vi "DFD Filter Array.vi"(7 "init (F)":bool, 8 "error in (no error)":errorcluster, 10 "filters":T1[](array[typedef]) {"mSRate_QSettings"."source" items=["Coef a/k"=0, "Coef b/v"=7, "Input"=1, "Output"=2, "Multiplicand"=3, "Product"=4, "Sum"=5, "Delay"=6, "Gain"=8]}, 11 "signal in":waveform(dbl)[](array[waveform])) -> (0 "error out":errorcluster, 3 "signal out":waveform(dbl)[](array[waveform]))   [LabVIEW 2019, in "Instrument.Lockin.lvlib" / "Instrument.DAQ.lvclass"]
uses:
  Instrument.DAQ.lvclass
  <vilib>/addons/Digital Filter Design/NI_DigFilterLicensed.lvlib
  <vilib>/addons/Digital Filter Design/NI_DigFilter_Process.lvlib
  <vilib>/addons/Digital Filter Design/Process.llb/DFD Filtering with State (Wfm).vi
  <vilib>/addons/Digital Filter Design/_Objects.llb/DFD Filter Structure Type Selector.ctl
  <vilib>/addons/Digital Filter Design/_Objects.llb/DFD Filter Coef.ctl
  <vilib>/addons/Digital Filter Design/_Objects.llb/dfd_Internal Quantization Srcs.ctl
  <vilib>/addons/Digital Filter Design/_Objects.llb/dfd_Internal Quantization Settings.ctl
  <vilib>/addons/Digital Filter Design/_Objects.llb/DFD Coef Norm Type.ctl
  <vilib>/addons/Digital Filter Design/_Objects.llb/DFD Filter Obj.ctl
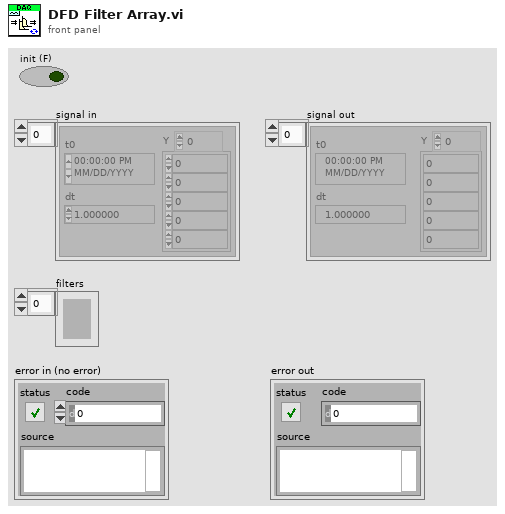
[diagram p1: front panel]
types:
  T1 = typedef "NI_DigFilterLicensed.lvlib/DFD Filter Obj.ctl" = cluster{"mSRate_Fs":dbl, "mSRate_Version":string, "mSRate_Comments":string, "mSRate_OrgCoef":T2, "mSRate_CurCoef":T2, "mSRate_Quantized?":bool, "mSRate_QCoef":T2, "mSRate_QSettings":T4[], "mSRate_Order":i32, "mSRate_Scaling":cluster{"mSRate_ScaleByPowerOf2?":bool, "mSRate_ScaleType":T6}}
  T2 = typedef "NI_DigFilterLicensed.lvlib/DFD Filter Coef.ctl" = cluster{"type":T3, "gain":dbl, "coef a (k)":dbl[], "coef b (v)":dbl[]}
  T3 = typedef "NI_DigFilterLicensed.lvlib/DFD Filter Structure Type Selector.ctl" = enum16{"Undefined", "FIR Direct Form", "FIR Direct Form Transposed", "FIR Symmetric", "FIR Antisymmetric", "IIR Direct Form I", "IIR Direct Form I Transposed", "IIR Direct Form II", "IIR Direct Form II Transposed", "IIR Cascaded Second Order Sections Form I", "IIR Cascaded Second Order Sections Form I Transposed", "IIR Cascaded Second Order Sections Form II", "IIR Cascaded Second Order Sections Form II Transposed", "Lattice Allpass (basic sections)", "Lattice Allpass (one multiplier sections)", "Lattice Allpass (normalized sections)", "Lattice AR (basic sections)", "Lattice AR (one multiplier sections)", "Lattice AR (normalized sections)", "Lattice MA (minimum phase)", "Lattice MA (maximum phase)", "Lattice ARMA (basic sections)", "Lattice ARMA (one multiplier sections)", "Lattice ARMA (normalized sections)"}
  T4 = typedef "NI_DigFilterLicensed.lvlib/dfd_Internal Quantization Settings.ctl" = cluster{"source":T5, "wl":i16, "iwl":i16, "overflow mode":enum16{"Saturation", "Wrap"}, "rounding mode":enum16{"Nearest", "Truncation"}, "signed?":bool}
  T5 = typedef "NI_DigFilterLicensed.lvlib/dfd_Internal Quantization Srcs.ctl" = u16
  T6 = typedef "NI_DigFilterLicensed.lvlib/DFD Coef Norm Type.ctl" = enum16{"No Norm", "Time Domain 1-Norm", "Time Domain 2-Norm", "Time Domain Inf-Norm"}
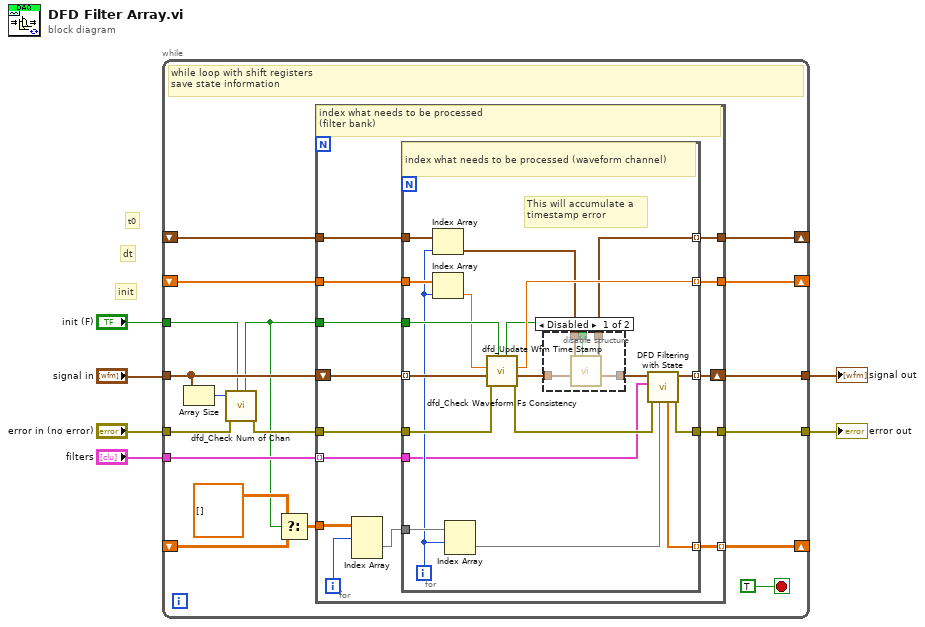
[diagram p0: block diagram]
diagram:
  # "t0"
  # "dt"
  # "init"
  n1 = while {
    tunnel: "init (F)" -> [w10]
    tunnel: "filters" -> [w22]
    shift-right: [w20] -> _
    shift-left: _ -> [w19]
    tunnel: "error in (no error)" -> [w8]
    tunnel: [w23] -> w2
    tunnel: "signal in" -> [w11]
    tunnel: [w24] -> w1
    shift-right: [w15] -> _
    shift-left: _ -> [w13]
    shift-right: [w16] -> _
    shift-left: _ -> [w14]
    stop <- TRUE stop-if-true
    # "while loop with shift registers \nsave state information"
    n2 = Array Size(array=w11) -> (size(s)=w12:i32)
    n3 = call <vilib>:"dfd_Check Num of Chan.vi"("init in"=w10, "error in (no error)"=w8, "#ch in"=w12) -> ("error out"=w9:errorcluster, "init out"=w7:bool)  [unwired: 7 out]
    n4 = Select(t=dbl[][][] [], s=w7, f=w19) -> (s? t:f=w17:dbl[][][])
    n5 = for {
      tunnel: w22 -> [w34] mode=indexing
      tunnel: [w33] -> w20 mode=indexing
      tunnel: w9 -> [w36]
      tunnel: [w37] -> w23
      tunnel: w17 -> [w32]
      tunnel: w7 -> [w29]
      shift-right: [w38] -> w24
      shift-left: w11 -> [w35]
      tunnel: [w28] -> w16
      tunnel: [w27] -> w15
      tunnel: w14 -> [w26]
      tunnel: w13 -> [w25]
      i -> [w31]
      # "index what needs to be processed\n(filter bank)"
      n6 = Index Array(array=w32, index (dim 0)=w31) -> (element=w30:dbl[][])  [unwired: 2 in]
      n7 = for {
        tunnel: [w58] -> w33 mode=indexing
        tunnel: w30 -> [w57]
        tunnel: w34 -> [w46]
        tunnel: w36 -> [w53]
        tunnel: [w39] -> w37
        tunnel: w35 -> [w55] mode=indexing
        tunnel: [w43] -> w38 mode=indexing
        tunnel: w29 -> [w52]
        tunnel: [w51] -> w27 mode=indexing
        tunnel: [w42] -> w28 mode=indexing
        tunnel: w26 -> [w50]
        tunnel: w25 -> [w49]
        i -> [w47]
        # "This will accumulate a \ntimestamp error"
        # "index what needs to be processed (waveform channel)"
        n8 = Index Array(array=w50, index=w47) -> (element=w44:timestamp)
        n9 = Index Array(array=w49, index=w47) -> (element=w45:dbl)
        n10 = Index Array(array=w57, index (row)=w47) -> (element=w56:dbl[])  [unwired: 1 in]
        n11 = call <vilib>:"dfd_Check Waveform Fs Consistency.vi"("init in"=w52, "error in (no error)"=w53, "signal in"=w55, "dt in"=w45) -> ("error out"=w54:errorcluster, "signal out"=w41:waveform(dbl), "dt out"=w51:dbl, "init out"=w48:bool)  [unwired: 4 out]
        n12 = disable-structure shown="Disabled" {
          disable-tunnel: w48 -> [w63 _]
          disable-tunnel: w44 -> [w62 _]
          disable-tunnel: [w61 _] -> w42
          disable-tunnel: w41 -> [w60 w64]
          disable-tunnel: [w59 w64] -> w40
          frame Disabled {
            n13 = call <vilib>:"dfd_Update Wfm Time Stamp.vi"("init? (F)"=w63, "signal in"=w60, "t0"=w62) -> ("signal out"=w59:waveform(dbl), "tf"=w61:timestamp)  [unwired: 1 in, 6 out]
          }
          frame Enabled {
          }
        }
        n14 = call-poly <vilib>:"DFD Filtering with State.vi"("state in"=w56, "error in (no error)"=w54, "filter"=w46, "signal in"=w40) -> ("error out"=w39:errorcluster, "signal out"=w43:waveform(dbl), "state out"=w58:dbl[])  [unwired: 5 in]
      }
    }
  }
  "error out" <- w2
  "signal out" <- w1
